vi "SplitFileStringProj2.vi"(0 "String from file":string) -> (4 "output cluster":T1, 12 "Frequency (Hz)":dbl[](array[numeric]), 13 "Amplitude (V)":dbl[](array[numeric]), 14 "Pøenos (dB)":dbl[](array[numeric]))   [LabVIEW 2021]
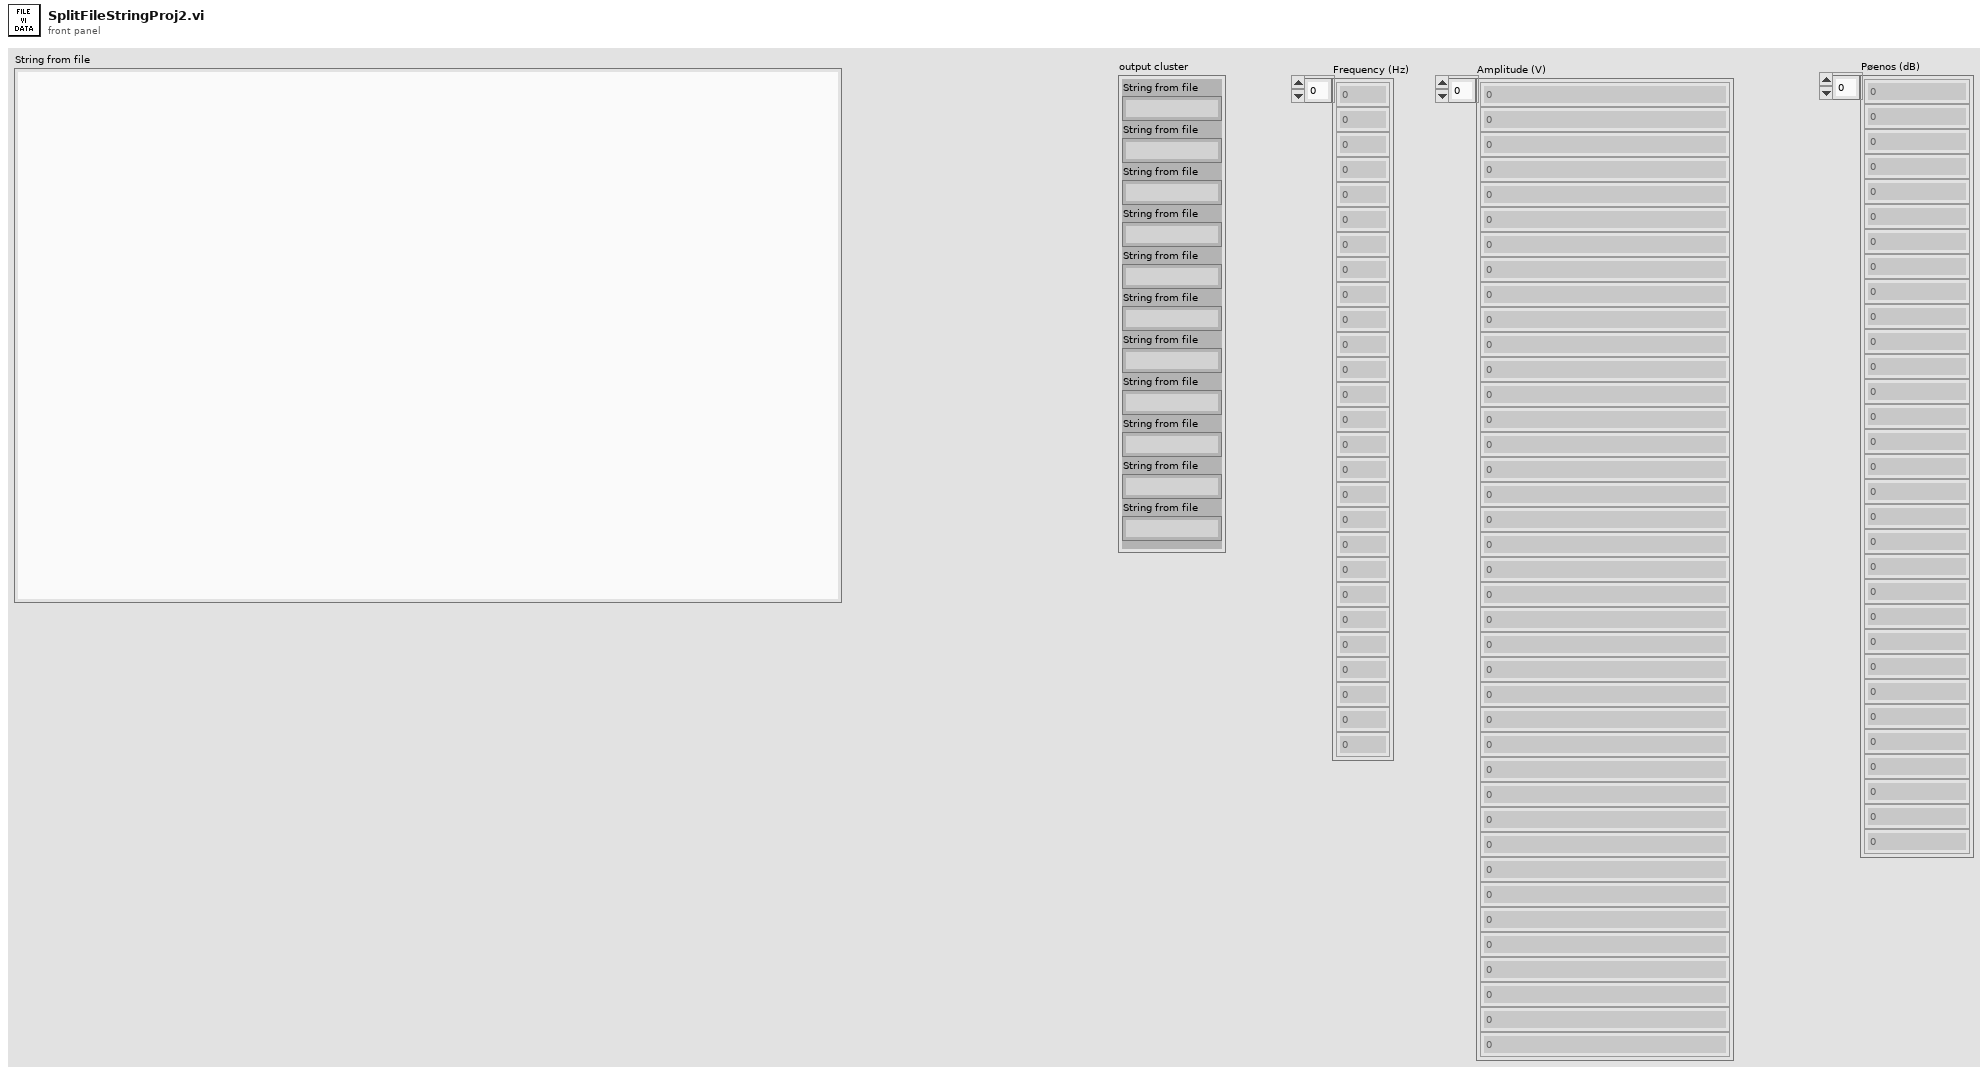
[diagram p1: front panel]
types:
  T1 = cluster{"String from file":string, "String from file":string, "String from file":string, "String from file":string, "String from file":string, "String from file":string, "String from file":string, "String from file":string, "String from file":string, "String from file":string, "String from file":string}
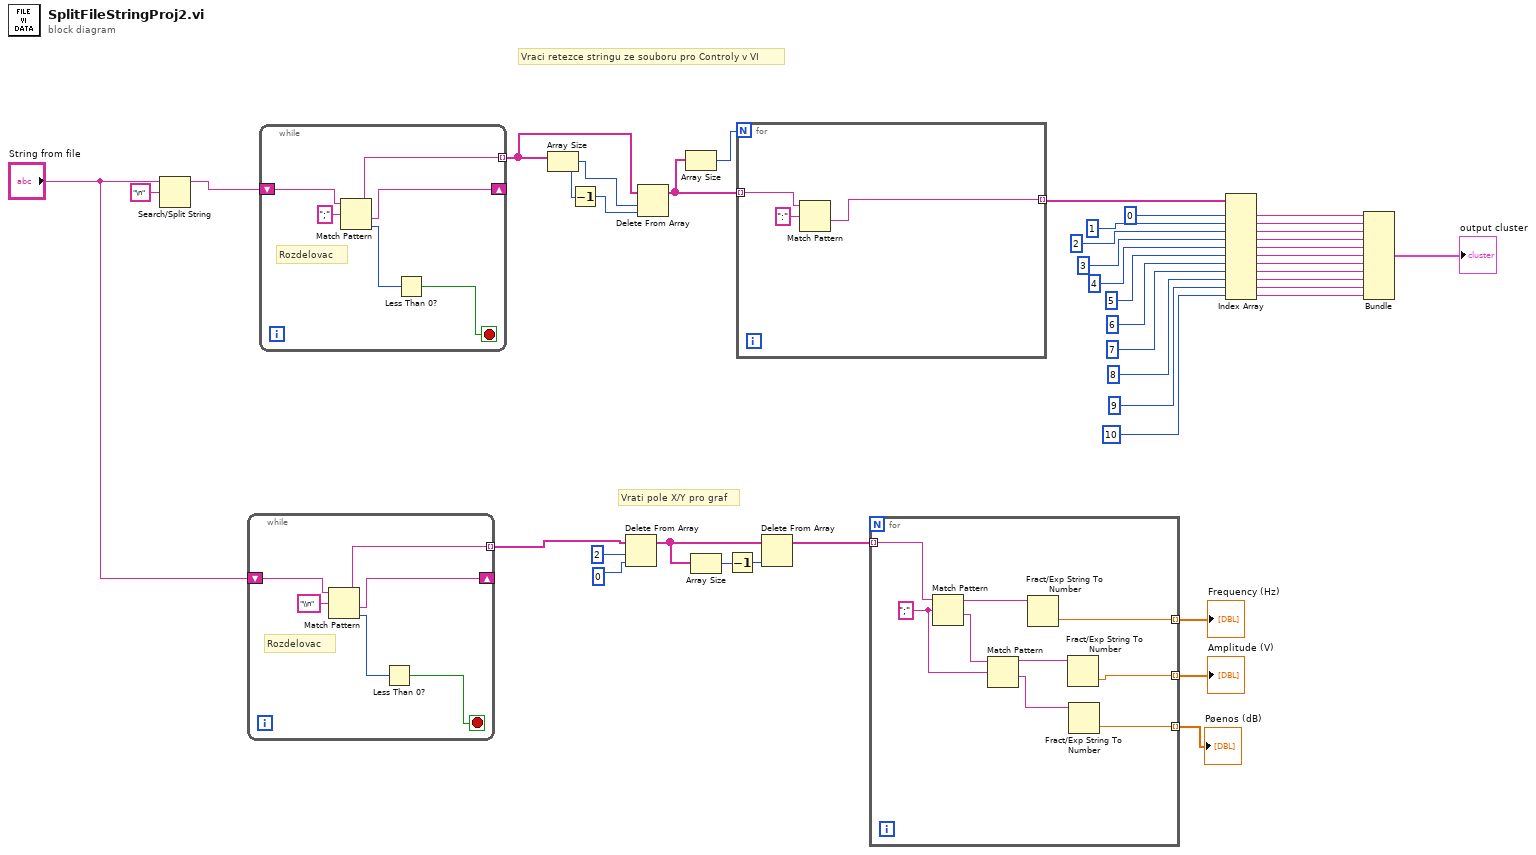
[diagram p0: block diagram]
diagram:
  # "Vrati pole X/Y pro graf"
  # "Vraci retezce stringu ze souboru pro Controly v VI"
  n1 = Search/Split String(string="String from file", search string/char (-)="\n") -> (substring before match=w29:string)  [unwired: 1 in, 2 out]
  n2 = while {
    shift-right: [w44] -> _
    shift-left: "String from file" -> [w45]
    tunnel: [w43] -> w25 mode=indexing
    stop <- w46 stop-if-true
    # "Rozdelovac"
    n3 = Match Pattern(string=w45, regular expression="\\n") -> (before substring=w43:string, after substring=w44:string, offset past match=w47:i32)  [unwired: 1 in, 1 out]
    n4 = Less Than 0?(x=w47) -> (x < 0?=w46:bool)
  }
  n5 = while {
    shift-right: [w50] -> _
    shift-left: w29 -> [w51]
    tunnel: [w49] -> w40 mode=indexing
    stop <- w52 stop-if-true
    # "Rozdelovac"
    n6 = Match Pattern(string=w51, regular expression=";") -> (before substring=w49:string, after substring=w50:string, offset past match=w53:i32)  [unwired: 1 in, 1 out]
    n7 = Less Than 0?(x=w53) -> (x < 0?=w52:bool)
  }
  n8 = Array Size(array=w40) -> (size(s)=w39:i32)
  n9 = Decrement(x=w39) -> (x-1=w41:i32)
  n10 = Delete From Array(array=w25, length=2, index=0) -> (array with subset deleted=w22:string[])  [unwired: 1 out]
  n11 = Delete From Array(array=w40, length=w39, index=w41) -> (array with subset deleted=w37:string[])  [unwired: 1 out]
  n12 = Array Size(array=w37) -> (size(s)=w38:i32)
  n13 = Array Size(array=w22) -> (size(s)=w24:i32)
  n14 = Decrement(x=w24) -> (x-1=w23:i32)
  n15 = for {
    N: w38 -> [_]
    tunnel: w37 -> [w57] mode=indexing
    tunnel: [w55] -> w36 mode=indexing
    n16 = Match Pattern(string=w57, regular expression=":") -> (after substring=w55:string)  [unwired: 1 in, 3 out]
  }
  n17 = Delete From Array(array=w22, index=w23) -> (array with subset deleted=w21:string[])  [unwired: 1 in, 1 out]
  n18 = for {
    tunnel: w21 -> [w66] mode=indexing
    tunnel: [w64] -> w20 mode=indexing
    tunnel: [w60] -> w19 mode=indexing
    tunnel: [w58] -> w18 mode=indexing
    w63 = ";" ("regular expression")
    n19 = Match Pattern(string=w66, regular expression=w63) -> (before substring=w65:string, after substring=w62:string)  [unwired: 1 in, 2 out]
    n20 = Match Pattern(string=w62, regular expression=w63) -> (before substring=w61:string, after substring=w59:string)  [unwired: 1 in, 2 out]
    n21 = Fract/Exp String To Number(string=w65) -> (number=w64:dbl)  [unwired: 3 in, 1 out]
    n22 = Fract/Exp String To Number(string=w61) -> (number=w60:dbl)  [unwired: 3 in, 1 out]
    n23 = Fract/Exp String To Number(string=w59) -> (number=w58:dbl)  [unwired: 3 in, 1 out]
  }
  "Frequency (Hz)" <- w20
  "Amplitude (V)" <- w19
  "Pøenos (dB)" <- w18
  n24 = Index Array(array=w36, index #1=0 ("index"), index #2=1 ("index"), index #3=2 ("index"), index #4=3 ("index"), index #5=4 ("index"), index #6=5 ("index"), index #7=6 ("index"), index #8=7 ("index"), index #9=8 ("index"), index #10=9 ("index"), index #11=10 ("index")) -> (element #1=w17:string, element #2=w16:string, element #3=w10:string, element #4=w9:string, element #5=w8:string, element #6=w7:string, element #7=w6:string, element #8=w5:string, element #9=w4:string, element #10=w3:string, element #11=w2:string)
  n25 = Bundle("String from file"=w17, "String from file"=w16, "String from file"=w10, "String from file"=w9, "String from file"=w8, "String from file"=w7, "String from file"=w6, "String from file"=w5, "String from file"=w4, "String from file"=w3, "String from file"=w2) -> (→"output cluster":T1)  [unwired: 1 in]
